vi "dat_pressure_sensors.vi"() -> (0 "P_lp2":fxp<+/-,24,5>, 1 "P_lp1":fxp<+/-,24,5>, 2 "P_hp2":fxp<+/-,24,5>, 3 "P_hp1":fxp<+/-,24,5>)   [LabVIEW 2018]
uses:
  <vilib>/rvi/Emulation/niFpgaEmulationIsFPGAContextNoSignature.vi
  <vilib>/rvi/DataTransferAndStorage/Container/Common/niFpgaContainerGetUniqueNameForEmu.vi
  <vilib>/rvi/Memory/Memory_Emulation/niFpgaMemoryEmulationCacheClearOnFirstRun.vi
  <vilib>/rvi/Memory/Memory_Emulation/nirvimemoryEmulationManagerCache_MakeExclusive.vi
  <vilib>/rvi/Memory/Memory_Emulation/niFpgaMemoryEmulationValidateCache.vi
  <vilib>/rvi/Memory/Memory_Emulation/nirvimemoryEmulationManagerCache_InsertValue.vi
  <vilib>/Utility/error.llb/Clear Errors.vi
  <vilib>/rvi/Memory/Memory_Emulation/nirvimemoryEmulationManagerCache_ReleaseExclusive.vi
  <vilib>/rvi/Memory/Memory_Emulation/nirvimemoryEmulationManagerCache_GetValue.vi
  <vilib>/rvi/Memory/Memory_Emulation/nirvimemoryEmulationManagerCache_SetValue.vi
  <vilib>/rvi/Emulation/niFpgaProcessEmulError.vi
  <vilib>/rvi/Emulation/niFpgaSctlEmulationGetInTimedLoop.vi
  <vilib>/rvi/DataTransferAndStorage/Container/XNode/niFpgaContainer.xnode
  <vilib>/rvi/DataTransferAndStorage/Register/Emulation/niFpgaRegisterEmulation.vi
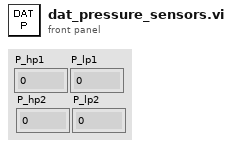
[diagram p1: front panel]
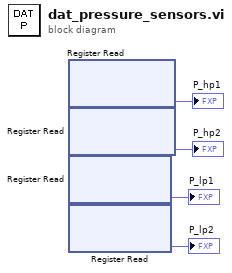
[diagram p0: block diagram]
diagram:
  n1 = xnode "Register Read"() -> ("Data"=→"P_hp1":fxp<+/-,24,5>)  [unwired: 1 in, 1 out]
  n2 = xnode "Register Read"() -> ("Data"=→"P_hp2":fxp<+/-,24,5>)  [unwired: 1 in, 1 out]
  n3 = xnode "Register Read"() -> ("Data"=→"P_lp1":fxp<+/-,24,5>)  [unwired: 1 in, 1 out]
  n4 = xnode "Register Read"() -> ("Data"=→"P_lp2":fxp<+/-,24,5>)  [unwired: 1 in, 1 out]
